vi "Correct_Scani_Valve_Pos.vi"() -> ()   [LabVIEW 2011]
panel:
  in  "Folder of RD Folders":path
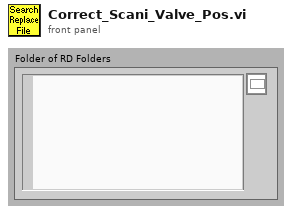
[diagram p1: front panel]
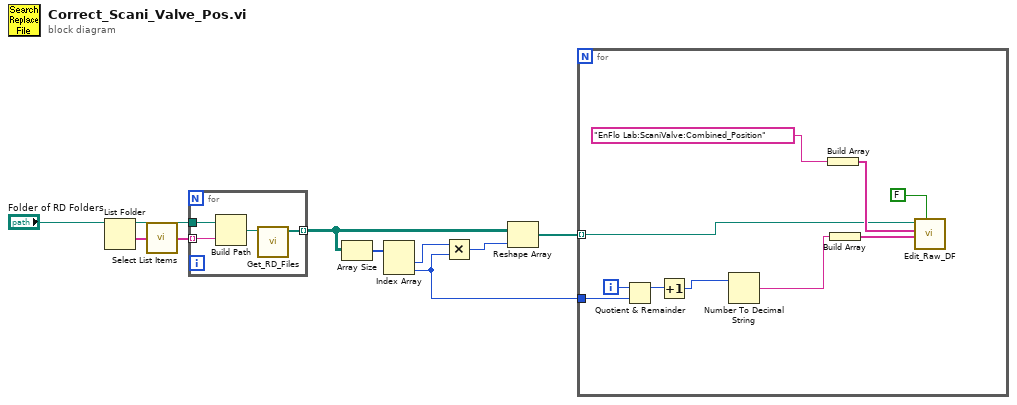
[diagram p0: block diagram]
diagram:
  n1 = List Folder(path="Folder of RD Folders") -> (path out=w8:path, folder names=w9:string[])  [unwired: 3 in, 2 out]
  n2 = call "Select List Items.vi"("Item Names"=w9) -> ("Selected Items"=w7:string[])  [unwired: 4 in]
  n3 = for {
    tunnel: w8 -> [w13]
    tunnel: w7 -> [w12] mode=indexing
    tunnel: [w11] -> w3 mode=indexing
    n4 = Build Path(base path=w13, name or relative path=w12) -> (appended path=w14:path)
    n5 = call "Get_RD_Files.vi"("Raw Data File Folder"=w14) -> ("Array of only RD Files"=w11:path[])  [unwired: 10 in]
  }
  n6 = Array Size(array=w3) -> (size(s)=w4:i32[])
  n7 = Index Array(array=w4) -> (element #1=w5:i32, element #2=w1:i32)  [unwired: 2 in]
  n8 = Multiply(x=w5, y=w1) -> (x*y=w6:i32)
  n9 = Reshape Array(w3, w6) -> (w2:path[])
  n10 = for {
    tunnel: w2 -> [w16] mode=indexing
    tunnel: w1 -> [w23]
    i -> [w24]
    n11 = Quotient & Remainder(x=w24, y=w23) -> (x-y*floor(x/y)=w22:i32)  [unwired: 1 out]
    n12 = Increment(x=w22) -> (x+1=w19:i32)
    n13 = Number To Decimal String(number=w19) -> (decimal integer string=w18:string)  [unwired: 1 in]
    n14 = Build Array("EnFlo Lab:ScaniValve:Combined_Position") -> (w20:string[])
    n15 = Build Array(w18) -> (w17:string[])
    n16 = call "Edit_Raw_DF.vi"("Edit Raw Data Header Info"=FALSE, "New Values In"=w17, "New Chs In"=w20, "Data filename"=w16) -> ()  [unwired: 2 in, 4 out]
  }
